vi "AuMT8852B Tester Authenticate.vi"(5 "Authentication On? (False)":bool=TRUE caption="Authentication State (OFF)", 7 "Set/Get (Set)":enum16{"Set", "Get"}(ring), 8 "error in (no error)":errorcluster, 11 "VISA session":refnum<visa-resource-name>) -> (0 "error out":errorcluster, 2 "error code":i32, 3 "VISA session out":refnum<visa-resource-name>, 4 "Authentication State out":bool=TRUE)   [LabVIEW 2017]
doc: "Anritsu MT8852B Bluetooth Tester\n\nControls the connection authentication state.\n\nINPUTS\nSet/Get - whether the value is being sent to or retrieved from the instrument.\nAuthentication State - enables or disables the connection authentication.\n\nOUTPUTS\nAuthentication State out - the current state of connection authentication."
uses:
  <instrlib>/aumt8852B/General/Utilities/MT8850 Attribute ID.ctl
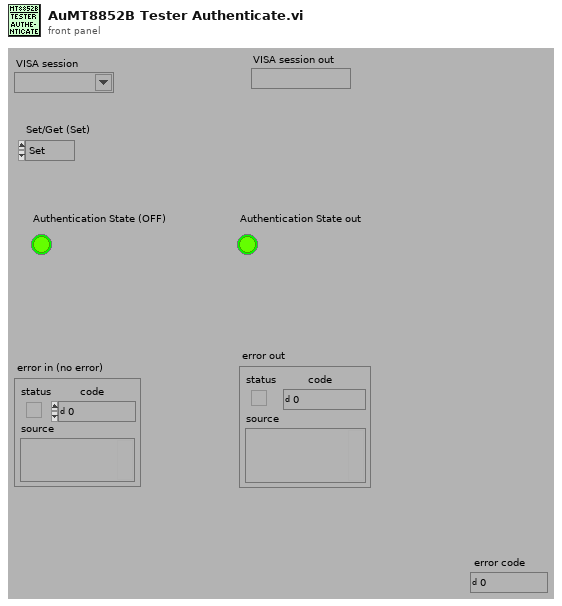
[diagram p1: front panel]
types:
  T1 = typedef "MT8850 Attribute ID.ctl" = enum16{"Operation mode", "Selected script", "EUT address source", "EUT Address", "EUT HCI RS232 Baud Rate", "Tester GPIB Address", "Tester RS232 Baud Rate", "Tester Bluetooth Address", "Tester Contrast", "Tester Key Click On", "Tester Modulation Index", "Tester Poll-Null Mode", "Tester Power Range", "Tester RS232 Mode", "Beep on Illegal Entry", "Display User Text", "User Text", "Calibration TX Modulation DAC", "Calibration RX Channel", "Calibration TX Channel", "Calibration TX Power", "Calibration Use TX Table", "Inquiry Request User-friendly Name", "Inquiry Number of Responses", "Inquiry Timeout", "Script Frequency Display", "Script Loop Count", "Script Loop Continuously", "Script Loop Stop on Fail", "Link timeout", "Page timeout", "Filter bandwidth", "SCO air code", "SCO bit position", "SCO input code", "SCO input data", "SCO input sample size", "SCO loopback mode", "SCO packet type", "SCO tone generator", "Tester page scan repetition mode", "Tester follow test mode", "Tester authentication state", "Tester authentication pin code", "Tester authentication pin length"}
  T2 = typedef "Attribute Status.ctl" = enum16{"No I/O needed", "I/O needed"}
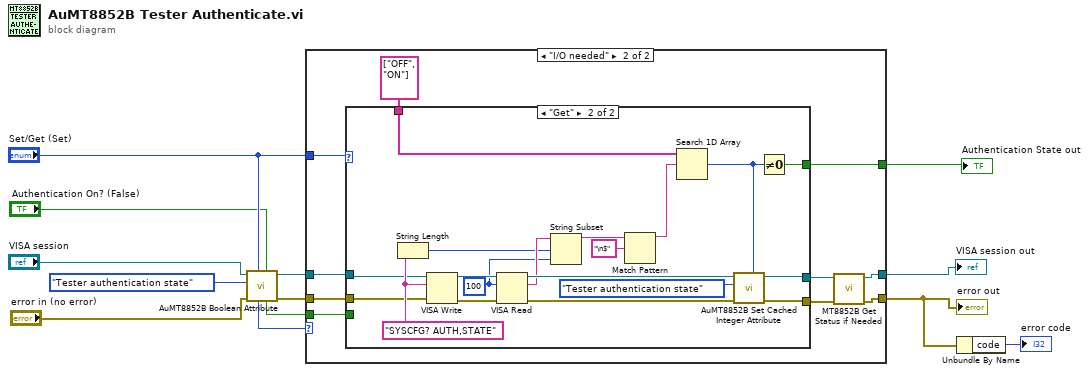
[diagram p0: block diagram]
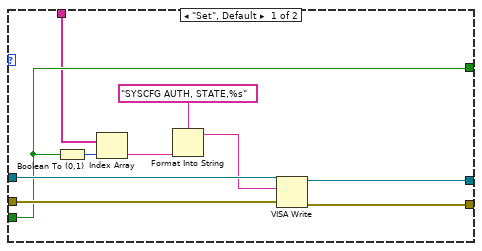
[diagram p3: hidden frame]
diagram:
  n1 = call <instrlib>:"AuMT8852B Boolean Attribute.vi"("Value (F)"="Authentication On? (False)", "Set/Get (Set)"="Set/Get (Set)", "error in (no error)"="error in (no error)", "Attribute ID"=MT8850_Attribute_ID."Tester authentication state", "VISA session"="VISA session") -> ("error out"=w4:errorcluster, "VISA session out"=w3:refnum<visa-resource-name>, "Value out"=w6:bool, "Status"=w8:T2)  [unwired: 3 in]
  n2 = case shown="\"I/O needed\"" w8 {
    tunnel: [w14 w25] -> w13
    tunnel: [w15 w26] -> w1
    tunnel: "Set/Get (Set)" -> [_ w22]
    tunnel: w6 -> [w16 w18]
    tunnel: w4 -> [w15 w20]
    tunnel: w3 -> [w14 w19]
    tunnel: [w16 w17] -> w2
    frame "No I/O needed", Default {
    }
    frame "I/O needed" {
      n3 = case shown="\"Get\"" w22 {
        tunnel: [w27 w39] -> w23
        tunnel: [w28 w40] -> w24
        tunnel: string[] ["OFF", "ON"] -> [w30 w38]
        tunnel: w20 -> [w36 w42]
        tunnel: w19 -> [w35 w41]
        tunnel: [w32 w37] -> w17
        tunnel: w18 -> [w32 _]
        frame "Set", Default {
          n4 = Boolean To (0,1)(Boolean=w32) -> (0, 1=w33:i16)
          n5 = Index Array(array=w30, index=w33) -> (element=w34:string)
          n6 = Format Into String(format string="SYSCFG AUTH, STATE,%s", w34) -> (resulting string=w29:string)  [unwired: 2 in, 1 out]
          n7 = VISA Write(VISA resource name=w35, write buffer=w29, error in (no error)=w36) -> (VISA resource name out=w27:refnum<visa-resource-name>, error out=w28:errorcluster)  [unwired: 1 out]
        }
        frame "Get" {
          w43 = u32 100 ("byte count (0)")
          w48 = "SYSCFG? AUTH,STATE" ("write buffer (\"\")")
          n8 = String Length(string=w48) -> (length=w47:i32)
          n9 = VISA Write(VISA resource name=w41, write buffer=w48, error in (no error)=w42) -> (VISA resource name out=w55:refnum<visa-resource-name>, error out=w54:errorcluster)  [unwired: 1 out]
          n10 = VISA Read(VISA resource name=w55, byte count=w43, error in (no error)=w54) -> (VISA resource name out=w53:refnum<visa-resource-name>, read buffer=w50:string, error out=w52:errorcluster)  [unwired: 1 out]
          n11 = String Subset(string=w50, offset (0)=w47, length (rest)=w43) -> (substring=w45:string)
          n12 = Match Pattern(string=w45, regular expression="\n$") -> (before substring=w46:string)  [unwired: 1 in, 3 out]
          n13 = Search 1D Array(1D array=w38, element=w46) -> (index of element=w49:i32)  [unwired: 1 in]
          n14 = call <instrlib>:"AuMT8852B Set Cached Integer Attribute.vi"("Value (0)"=w49, "error in (no error)"=w52, "Attribute ID"=MT8850_Attribute_ID."Tester authentication state", "VISA session"=w53) -> ("error out"=w40:errorcluster, "VISA session out"=w39:refnum<visa-resource-name>)  [unwired: 6 in]
          n15 = Not Equal To 0?(x=w49) -> (x != 0?=w37:bool)
        }
      }
      n16 = call <instrlib>:"MT8852B Get Status if Needed.vi"("error in (no error)"=w24, "VISA session"=w23) -> ("error out"=w26:errorcluster, "VISA session out"=w25:refnum<visa-resource-name>)  [unwired: 8 in]
    }
  }
  "VISA session out" <- w13
  "error out" <- w1
  "Authentication State out" <- w2
  n17 = Unbundle By Name(w1) -> ("code"=→"error code":i32)
